vi "OscDataToWfm (SubVI).vi"(10 "Data":T1, 11 "A5000_param":T2={"ChannelA"={"Enabled"=FALSE, "Coupling"=0, "Range"=0, "Analogue Offset"=0.0}, "ChannelB"={"Enabled"=FALSE, "Coupling"=0, "Range"=0, "Analogue Offset"=0.0}, "Trigger"={"Trigger Enabled"=FALSE, "Trigger Source"=enum."Channel A", "Trigger Threshold (volts)"=0.0, "Trigger Direction"=0, "Trigger Delay (samples)"=0, "Auto Trigger Time (ms)"=0}, "MaxADCvalue"=0, "handle"=0, "Acquisition"={"preTriggerSamples"=0, "postTriggerSamples"=0, "timebase"=0, "Down-Sample Mode"=0, "Down Sample Ratio"=0}, "Device Info"={"Driver Version"="", "USB Version"="", "Hardware"="", "Variant"="", "Batch and Serial"="", "Cal Date"="", "Kernel Version"="", "Digital HW Version"="", "Analogue HW Version"="", "MSO"=FALSE, "Number of channels"=0}, "Properties"={"Sample Frequency"=0.0, "Sample Rate"=0.0, "Max Samples Available"=0, "Number of Samples"=0, "Total Capture Time (sec) "=0.0, "Max Total Capture Time Available (sec)"=0.0}, "Resolution"=0, "EmulateV"=FALSE, "General AWG Settings"={"Peak-to-Peak Voltage (microvolts)"=2000000, "Offset Voltage (microvolts)"=0, "Wave Type"=0, "Sweep Type"=0, "Shots"=0, "Sweeps"=0, "Trigger Type"=0, "Trigger Source"=0, "Ext. Threshold (ADC count)"=0, "White Noise/PRBS"=0}, "Standard Waveform Settings"={"Start Frequency"=1000.0, "Stop Frequency"=1000.0, "Increment"=0.0, "Dwell Time (seconds)"=0.0}, "Arbitrary Waveform Settings"={"Arbirary waveform file path"=path "", "Index Mode"=0}} {"Arbitrary Waveform Settings"."Index Mode" items=["Single", "Dual", "Quad"]; "Standard Waveform Settings"."Stop Frequency" min=0.03 max=1000000.0; "Standard Waveform Settings"."Start Frequency" min=0.03 max=1000000.0; "General AWG Settings"."White Noise/PRBS" items=["Normal", "White Noise", "PRBS"]; "General AWG Settings"."Trigger Source" items=["None", "Scope Trigger", "Aux. In", "Ext. In", "Software Trigger"]; "General AWG Settings"."Trigger Type" items=["Rising", "Falling", "Gate High", "Gate Low"]; "General AWG Settings"."Sweep Type" items=["Up", "Down", "Up-Down", "Down-Up"]; "General AWG Settings"."Wave Type" items=["Sine", "Square", "Triangle", "Ramp Up", "Ramp Down", "Sinc", "Gaussian", "Half Sine", "DC", "Arbitrary"]; "Resolution" items=["8-bit", "12-bit", "14-bit", "15-bit (max. 2 ch.)", "16-bit (max. 1 ch.)"]; "Properties"."Max Total Capture Time Available (sec)" format="%.3p"; "Properties"."Sample Frequency" format="%.3p"; "Properties"."Sample Rate" format="%.3p"; "Properties"."Max Samples Available" format="%.3p"; "Properties"."Total Capture Time (sec)" format="%.3p"; "Acquisition"."Down Sample Ratio" min=1 step=1; "Acquisition"."Down-Sample Mode" items=["None"=0, "Aggregate"=1, "Decimate"=2, "Average"=4]; "Trigger"."Trigger Direction" items=["Rising"=2, "Falling"=3]; "ChannelB"."Range" items=["10 mV", "20 mV", "50 mV", "100 mV", "200 mV", "500 mV", "1 V", "2 V", "5 V", "10 V", "20 V"]; "ChannelB"."Coupling" items=["AC", "DC"]; "ChannelA"."Range" items=["10 mV", "20 mV", "50 mV", "100 mV", "200 mV", "500 mV", "1 V", "2 V", "5 V", "10 V", "20 V"]; "ChannelA"."Coupling" items=["AC", "DC"]}) -> (3 "Array":waveform(dbl)[](array[waveform]))   [LabVIEW 2017]
uses:
  controls/A5000_param.ctl
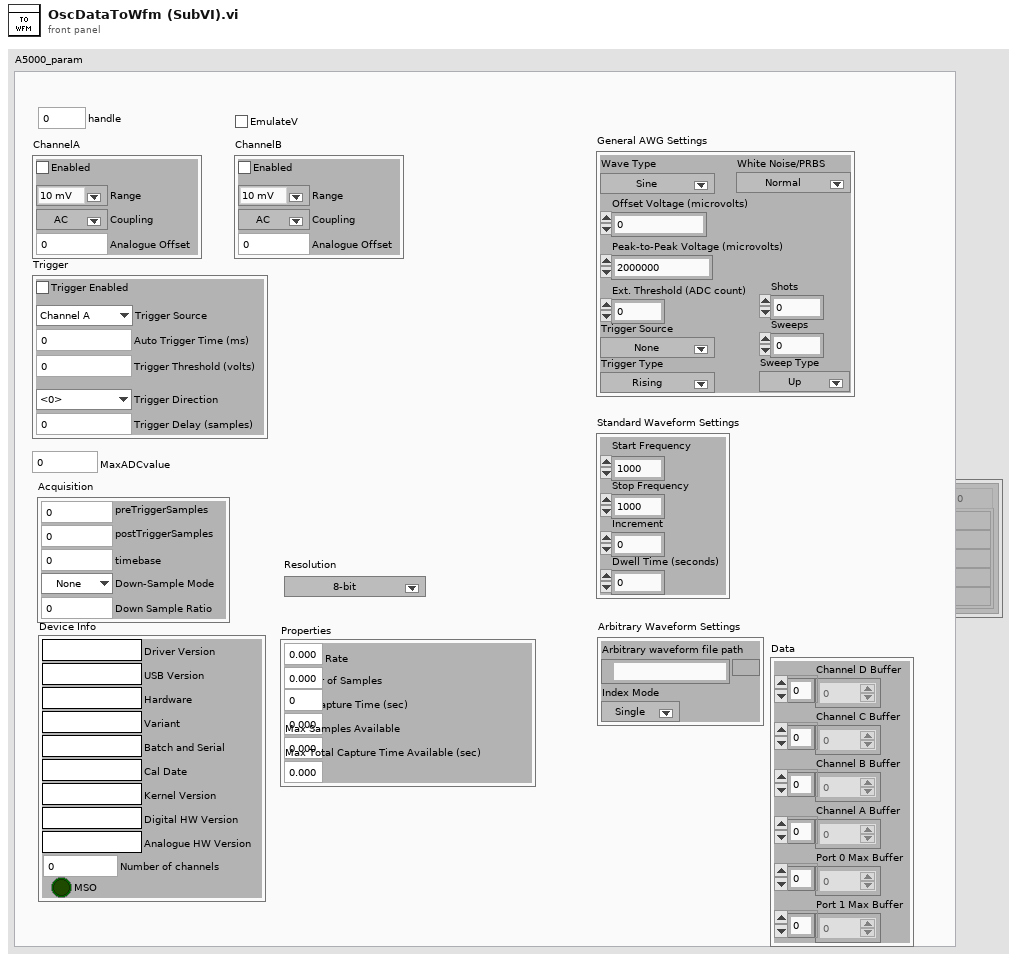
[diagram p1: front panel]
types:
  T1 = cluster{"Channel D Buffer":i16[], "Channel C Buffer":i16[], "Channel B Buffer":i16[], "Channel A Buffer":i16[], "Port 0 Max Buffer":i32[], "Port 1 Max Buffer":i32[]}
  T2 = typedef "A5000_param.ctl" = cluster{"ChannelA":cluster{"Enabled":bool, "Coupling":i16, "Range":u16, "Analogue Offset":sgl}, "ChannelB":cluster{"Enabled":bool, "Coupling":i16, "Range":u16, "Analogue Offset":sgl}, "Trigger":cluster{"Trigger Enabled":bool, "Trigger Source":enum16{"Channel A", "Channel B", "Channel C", "Channel D", "Ext."}, "Trigger Threshold (volts)":dbl, "Trigger Direction":u16, "Trigger Delay (samples)":u32, "Auto Trigger Time (ms)":i16}, "MaxADCvalue":i16, "handle":i16, "Acquisition":cluster{"preTriggerSamples":i32, "postTriggerSamples":i32, "timebase":u32, "Down-Sample Mode":u32, "Down Sample Ratio":u32}, "Device Info":cluster{"Driver Version":string, "USB Version":string, "Hardware":string, "Variant":string, "Batch and Serial":string, "Cal Date":string, "Kernel Version":string, "Digital HW Version":string, "Analogue HW Version":string, "MSO":bool, "Number of channels":i16}, "Properties":cluster{"Sample Frequency":sgl, "Sample Rate":sgl, "Max Samples Available":i32, "Number of Samples":u32, "Total Capture Time (sec) ":sgl, "Max Total Capture Time Available (sec)":sgl}, "Resolution":i32, "EmulateV":bool, "General AWG Settings":cluster{"Peak-to-Peak Voltage (microvolts)":u32, "Offset Voltage (microvolts)":i32, "Wave Type":u32, "Sweep Type":u32, "Shots":u32, "Sweeps":u32, "Trigger Type":u32, "Trigger Source":u32, "Ext. Threshold (ADC count)":i16, "White Noise/PRBS":u32}, "Standard Waveform Settings":cluster{"Start Frequency":dbl, "Stop Frequency":dbl, "Increment":dbl, "Dwell Time (seconds)":dbl}, "Arbitrary Waveform Settings":cluster{"Arbirary waveform file path":path, "Index Mode":u32}}
  T3 = cluster{"preTriggerSamples":i32, "postTriggerSamples":i32, "timebase":u32, "Down-Sample Mode":u32, "Down Sample Ratio":u32}
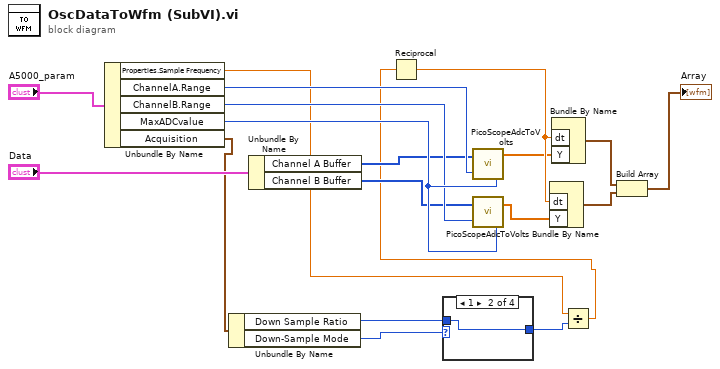
[diagram p0: block diagram]
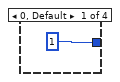
[diagram p2: hidden frame]
diagram:
  n1 = Unbundle By Name("A5000_param") -> ("Properties.Sample Frequency"=w3:sgl, "ChannelA.Range"=w11:u16, "ChannelB.Range"=w12:u16, "MaxADCvalue"=w19:i16, "Acquisition"=w4:T3)
  n2 = Unbundle By Name(w4) -> ("Down Sample Ratio"=w6:u32, "Down-Sample Mode"=w7:u32)
  n3 = Unbundle By Name("Data") -> ("Channel A Buffer"=w9:i16[], "Channel B Buffer"=w10:i16[])
  n4 = case shown="1" w7 {
    tunnel: w6 -> [_ w21 w22 w23]
    tunnel: [u32 1 ("Down Sample Ratio") w21 w22 w23] -> w2
    frame 0, Default {
    }
    frame 1 {
    }
    frame 2 {
    }
    frame 4 {
    }
  }
  n5 = call "PicoScopeAdcToVolts.vi"("Max_adc"=w19, "Range Index"=w11, "Data"=w9) -> ("Data (Volts)"=w13:dbl[])
  n6 = call "PicoScopeAdcToVolts.vi"("Max_adc"=w19, "Range Index"=w12, "Data"=w10) -> ("Data (Volts)"=w14:dbl[])
  n7 = Divide(x=w3, y=w2) -> (x/y=w1:sgl)
  n8 = Reciprocal(x=w1) -> (1/x=w15:sgl)
  n9 = Bundle By Name("dt"=w15, "Y"=w14) -> (w17:waveform(dbl))  [unwired: 1 in]
  n10 = Bundle By Name("dt"=w15, "Y"=w13) -> (w16:waveform(dbl))  [unwired: 1 in]
  n11 = Build Array(w16, w17) -> (→"Array":waveform(dbl)[])
